vi "Add User.vi"(0 "User Manager View in":refnum<class "User Manager View.lvclass">, 11 "error in (no error)":errorcluster) -> (4 "User Manager View out":refnum<class "User Manager View.lvclass">, 15 "error out":errorcluster)   [LabVIEW 2017, in "User Manager View.lvlib" / "User Manager View.lvclass"]
uses:
  <vilib>/gpm_packages/@cs/User Manager App/User Manager View/User Manager View/User Manager View.lvclass
  <vilib>/gpm_packages/@cs/User Manager App/User Manager View/User Manager Type Defs/State.ctl
  <vilib>/gpm_packages/@cs/User Manager App/User Manager View/User Manager View/User Manager View.lvclass/User Manager View.ctl
  <vilib>/gpm_packages/@cs/User Manager App/User Manager View/User Manager View.lvlib
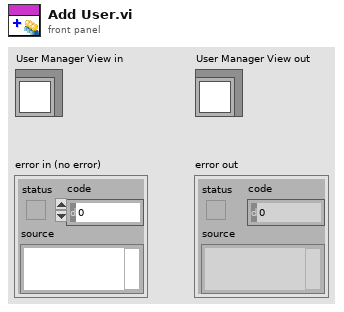
[diagram p1: front panel]
types:
  T1 = typedef "User Manager View.lvlib/State.ctl" = enum16{"Normal", "Adding User", "Changing User Data"}
  T2 = enum8{"Enabled", "Disabled", "Disabled and Grayed Out"}
  T3 = typedef "User Manager Application Types.lvlib/User Levels.ctl" = cluster{"Rank":i32, "Title":string}
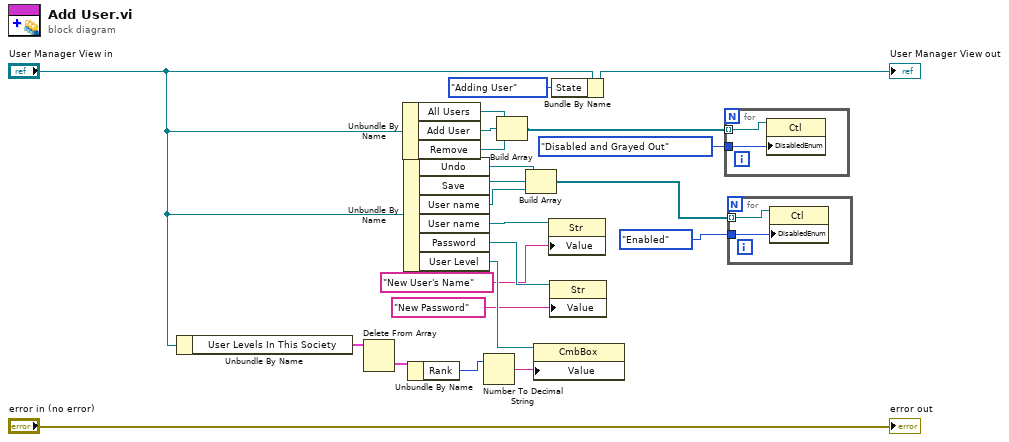
[diagram p0: block diagram]
diagram:
  n1 = Unbundle By Name("User Manager View in") -> ("User Levels In This Society"=w3:T3[])
  n2 = Delete From Array(array=w3) -> (deleted portion=w2:T3)  [unwired: 2 in, 1 out]
  n3 = Unbundle By Name("User Manager View in") -> ("All Users"=w20:refnum<vi>, "Add User"=w19:refnum<vi>, "Remove"=w12:refnum<vi>)
  n4 = Unbundle By Name("User Manager View in") -> ("Undo"=w15:refnum<vi>, "Save"=w14:refnum<vi>, "User name"=w11:refnum<vi>, "User name"=w10:refnum<vi>, "Password"=w9:refnum<vi>, "User Level"=w8:refnum<vi>)
  n5 = Unbundle By Name(w2) -> ("Rank"=w4:i32)
  n6 = Number To Decimal String(number=w4) -> (decimal integer string=w5:string)  [unwired: 1 in]
  n7 = Build Array(w20, w19, w12) -> (w18:refnum<vi>[])
  n8 = Build Array(w15, w14, w11) -> (w13:refnum<vi>[])
  n9 = property class="CmbBox"(reference=w8, "Value"=w5) -> ()  [unwired: 1 in, 2 out]
  n10 = property class="Str"(reference=w10, "Value"="New User's Name" ("User name")) -> ()  [unwired: 1 in, 2 out]
  n11 = property class="Str"(reference=w9, "Value"="New Password" ("Password")) -> ()  [unwired: 1 in, 2 out]
  n12 = Bundle By Name(cluster="User Manager View in", "State"=State."Adding User") -> (→"User Manager View out":refnum<class "User Manager View.lvclass">)
  n13 = for {
    tunnel: w18 -> [w25] mode=indexing
    tunnel: T2."Disabled and Grayed Out" ("Disabled") -> [w24]
    n14 = property class="Ctl"(reference=w25, "DisabledEnum"=w24) -> ()  [unwired: 1 in, 2 out]
  }
  n15 = for {
    tunnel: w13 -> [w27] mode=indexing
    tunnel: T2."Enabled" ("Disabled") -> [w26]
    n16 = property class="Ctl"(reference=w27, "DisabledEnum"=w26) -> ()  [unwired: 1 in, 2 out]
  }
  "error out" <- "error in (no error)"
